vi "Write X Scrollbar Visible.vi"(5 "X Scrollbar Visible":bool, 9 "GraphChart in":refnum<class "GraphChart.lvclass">) -> (3 "GraphChart out":refnum<class "GraphChart.lvclass">)   [LabVIEW 2014, in "GraphChart.lvclass"]
uses:
  GraphChart.lvclass
  GraphChart.lvclass/GraphChart.ctl
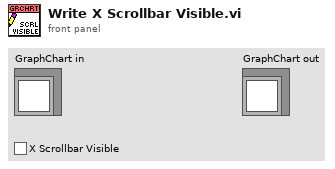
[diagram p1: front panel]
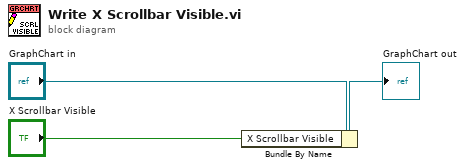
[diagram p0: block diagram]
diagram:
  n1 = Bundle By Name(cluster="GraphChart in", "X Scrollbar Visible"="X Scrollbar Visible") -> (→"GraphChart out":refnum<class "GraphChart.lvclass">)
